vi "no ramp right.vi"() -> ()   [LabVIEW 2012, in "Omni2013.lvrbt"]
uses:
  Omni2013.lvrbt
  <vilib>/NXT/Hardware/Plugins/Tetrix 180 deg Servo/Tetrix180ServoAddress.ctl
  <vilib>/NXT/Hardware/Plugins/Tetrix DC Motor/TetrixDCMotorAddress.ctl
  <vilib>/NXT/Block Support/NXT_InputPort.ctl
  <vilib>/NXT/HiTechnic/HiTechnic Controls/HiTechnic Port.ctl
  <vilib>/NXT/Dual Mode Library/Waits/Wait_Num(msec).vi
  <vilib>/NXT/NXTIO Xnodes/NXTIONodeSubVIs/TETRIX IO Move Servos.vi
  <vilib>/NXT/NXTIO Xnodes/NXTIONodeSubVIs/TETRIX IO Move DC Motors.vi
  <vilib>/NXT/HiTechnic/HiTechnic Config/HiTechnic IRSeeker Mode1200Hz.vi
  <vilib>/NXT/Dual Mode Library/Sensors/Sonar_cm.vi
  <vilib>/NXT/Dual Mode Library/Display/drawNumber.vi
  <vilib>/NXT/HiTechnic/HiTechnic Read/HiTechnic IRSeeker Sensor_DC all.vi
  <vilib>/NXT/NXTIO Xnodes/AddressXNode/NXTIOAddress.xnode
  <vilib>/NXT/NXTIO Xnodes/NXTIOXNode/NXTIO.xnode
  <vilib>/NXT/Subs/LVHSConnector.ctl
  <vilib>/NXT/LegoClasses/BrickReference/BrickReference.lvclass
panel:
  in  "Rotation":dbl
  in  "Translation L&R":dbl
  in  "Translation U&D":dbl
  in  "Initial Time":dbl
  out "Enabled":bool
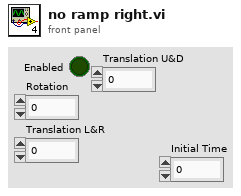
[diagram p1: front panel]
types:
  T1 = typedef "LVHSConnector.ctl" = refnum<class "BrickReference.lvclass">
  T2 = typedef "HiTechnic Port.ctl" = cluster{"Port":T3, "MUX Port":u8}
  T3 = typedef "NXT_InputPort.ctl" = u8
  T4 = typedef "TetrixDCMotorAddress.ctl" = i16
  T5 = cluster{"TetrixDCMotor":T4, "TetrixDCMotor 2":T4}
  T6 = typedef "Tetrix180ServoAddress.ctl" = i16
  T7 = cluster{"Direction (0-9)":i16, "Signal Strength (Array)":u8[]}
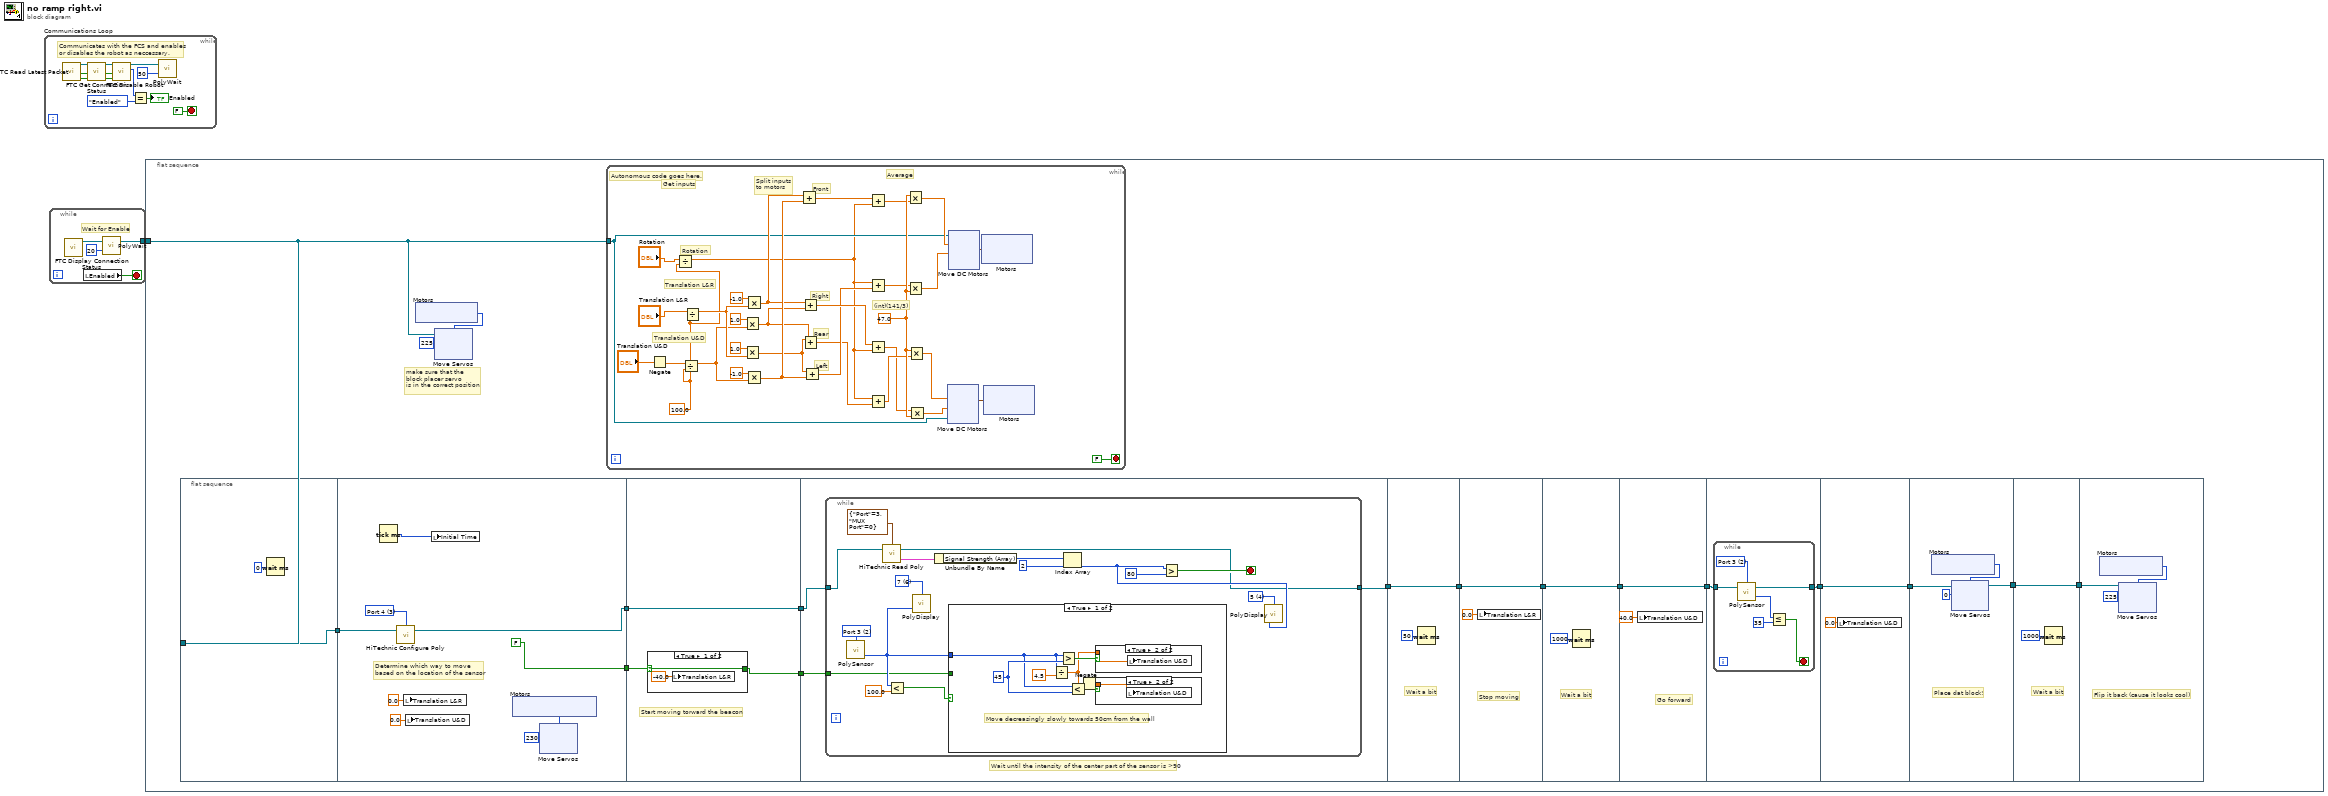
[diagram p0: block diagram]
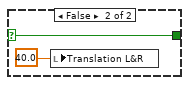
[diagram p2: hidden frame]
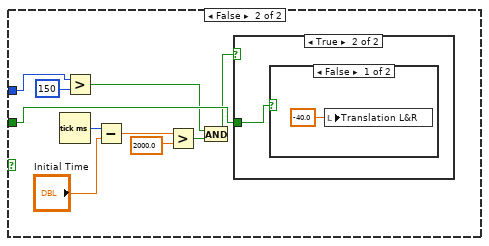
[diagram p5: hidden frame]
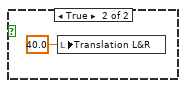
[diagram p7: hidden frame]
diagram:
  n1 = while "Communications Loop" {
    stop <- FALSE stop-if-true
    # "Communicates with the FCS and enables \nor disables the robot as neccessary."
    n2 = call <vilib>:"FTC Read Latest Packet.vi"() -> ("Packet Received?"=w11:bool, "Stopped?"=w10:bool, "NXT"=w13:T1)  [unwired: 6 in, 3 out]
    n3 = call <vilib>:"FTC Get Connection Status.vi"("Packet Received?"=w11, "Stopped?"=w10, "NXT"=w13) -> ("Online?"=w2:bool, "Stopped?"=w3:bool, "NXT"=w12:T1)  [unwired: 5 in]
    n4 = call <vilib>:"FTC Disable Robot.vi"("Online?"=w2, "Stopped?"=w3, "NXT"=w12) -> ("Enabled?"=w6:enum16{"Disabled", "Enabled"}, "NXT"=w8:T1)  [unwired: 3 in]
    n5 = Equal?(x=w6, y=enum16{"Disabled", "Enabled"}."Enabled") -> (x = y?=→"Enabled":bool)
    n6 = call-poly <vilib>:"PolyWait.vi"("Time (100 msec)"=u32 50 ("Time (msec)"), "NXT"=w8) -> ()  [unwired: 2 in, 1 out]
  }
  n7 = while {
    tunnel: [w15] -> w1
    stop <- w16 stop-if-true
    # "Wait for Enable"
    n8 = call <vilib>:"FTC Display Connection Status.vi"() -> ("NXT"=w14:T1)  [unwired: 11 in]
    n9 = local read "Enabled"() -> (w16:bool)
    n10 = call-poly <vilib>:"PolyWait.vi"("Time (100 msec)"=u32 20 ("Time (msec)"), "NXT"=w14) -> ("NXT"=w15:T1)  [unwired: 2 in]
  }
  n11 = flat-sequence {
    tunnel: w1 -> [w32]
    frame #0 {
      # "make sure that the \nblock placer servo \nis in the correct position"
      n12 = flat-sequence {
        tunnel: w32 -> [w44]
        tunnel: [w44] -> w18
        tunnel: [FALSE] -> w21
        tunnel: [w46] -> w20
        tunnel: w18 -> [w50]
        tunnel: [w64] -> w29
        tunnel: w21 -> [w63]
        tunnel: w20 -> [w64]
        tunnel: [w62] -> w19
        tunnel: w29 -> [w71]
        tunnel: [w70] -> w31
        tunnel: w19 -> [w69]
        tunnel: w31 -> [w111]
        tunnel: [w111] -> w30
        tunnel: [w112] -> w28
        tunnel: w30 -> [w112]
        tunnel: [w115] -> w22
        tunnel: w28 -> [w115]
        tunnel: w22 -> [w117]
        tunnel: [w117] -> w27
        tunnel: w27 -> [w119]
        tunnel: [w118] -> w26
        tunnel: w26 -> [w127]
        tunnel: [w127] -> w25
        tunnel: w25 -> [w129]
        tunnel: [w128] -> w24
        tunnel: w24 -> [w141]
        tunnel: [w141] -> w23
        tunnel: w23 -> [w142]
        frame #0 {
          n13 = Wait (ms)(milliseconds to wait=u32 0) -> ()  [unwired: 1 out]
        }
        frame #1 {
          w53 = T3 3 items=["Port 1", "Port 2", "Port 3", "Port 4"] ("Port")
          # "Determine which way to move \nbased on the location of the sensor"
          n14 = Tick Count (ms)() -> (millisecond timer value=w49:u32)
          n15 = call-poly <vilib>:"HiTechnic Configure Poly.vi"("NXT"=w50, "Port"=w53) -> ("NXT"=w46:T1)  [unwired: 2 in]
          n16 = local write "Translation L&R"(0.0 ("Translation L&R")) -> ()
          n17 = local write "Translation U&D"(0.0 ("Translation U&D")) -> ()
          n18 = local write "Initial Time"(w49) -> ()
          n19 = xnode "Motors"() -> ("Motor"=w48:T6)
          n20 = xnode "Move Servos"("Position 1"=u8 230, "Servos"=w48) -> ()  [unwired: 1 in, 1 out]
        }
        frame #2 {
          # "Start moving torward the beacon"
          n21 = case shown="True" w63 {
            selector: w63 -> [w65 w67]
            tunnel: [w65 w67] -> w62
            frame True {
              n22 = local write "Translation L&R"(-40.0 ("Translation L&R")) -> ()
            }
            frame False {
              n23 = local write "Translation L&R"(40.0 ("Translation L&R")) -> ()
            }
          }
        }
        frame #3 {
          # "Wait until the intensity of the center part of the sensor is >90"
          n24 = while {
            tunnel: w71 -> [w79]
            tunnel: [w77] -> w70
            tunnel: w69 -> [w72]
            stop <- w83 stop-if-true
            w76 = i16 6 items=["1", "2", "3", "4", "5", "6", "7", "8"] ("Line")
            w78 = T3 2 items=["Port 1", "Port 2", "Port 3", "Port 4"] ("Port (Port 4)")
            w82 = i16 4 items=["1", "2", "3", "4", "5", "6", "7", "8"] ("Line")
            n25 = call-poly <vilib>:"PolySensor.vi"("Port (Port 4)"=w78) -> ("Distance (cm)"=w74:i16)  [unwired: 2 in, 1 out]
            n26 = call-poly <vilib>:"HiTechnic Read Poly.vi"("NXT"=w79, "Port/MUX"=T2 {"Port"=3, "MUX Port"=0}) -> ("All Info"=w86:T7, "NXT"=w77:T1)  [unwired: 1 in]
            n27 = Less?(x=w74, y=100.0) -> (x < y?=w73:bool)
            n28 = call-poly <vilib>:"PolyDisplay.vi"("number"=w74, "Line"=w76) -> ()  [unwired: 2 in, 1 out]
            n29 = Unbundle By Name(w86) -> ("Signal Strength (Array)"=w85:u8[])
            n30 = case shown="True" w73 {
              tunnel: w74 -> [w90 w106]
              tunnel: w72 -> [_ w104]
              frame True {
                w92 = i16 45 ("y")
                # "Move decreasingly slowly towards 50cm from the wall"
                n31 = Divide(x=w90, y=4.5) -> (x/y=w89:dbl)
                n32 = Greater?(x=w90, y=w92) -> (0:w93:bool)
                n33 = Less?(x=w90, y=w92) -> (x < y?=w94:bool)
                n34 = Negate(x=w89) -> (-x=w88:dbl)
                n35 = case shown="True" w93 {
                  tunnel: w89 -> [_ w95]
                  frame False {
                  }
                  frame True {
                    n36 = local write "Translation U&D"(w95) -> ()
                  }
                }
                n37 = case shown="True" w94 {
                  tunnel: w88 -> [_ w96]
                  frame False {
                  }
                  frame True {
                    n38 = local write "Translation U&D"(w96) -> ()
                  }
                }
              }
              frame False {
                n39 = Tick Count (ms)() -> (millisecond timer value=w103:u32)
                n40 = Greater?(x=w106, y=i16 150) -> (0:w98:bool)
                n41 = Subtract(x=w103, y="Initial Time") -> (x-y=w101:dbl)
                n42 = Greater?(x=w101, y=2000.0) -> (0:w97:bool)
                n43 = And(x=w98, y=w97) -> (x .and. y?=w99:bool)
                n44 = case shown="True" w99 {
                  tunnel: w104 -> [_ w107]
                  frame False {
                  }
                  frame True {
                    n45 = case shown="False" w107 {
                      frame False {
                        n46 = local write "Translation L&R"(-40.0 ("Translation L&R")) -> ()
                      }
                      frame True {
                        n47 = local write "Translation L&R"(40.0 ("Translation L&R")) -> ()
                      }
                    }
                  }
                }
              }
            }
            n48 = Index Array(array=w85, index=2) -> (element=w81:u8)
            n49 = Greater?(x=w81, y=u8 80) -> (0:w83:bool)
            n50 = call-poly <vilib>:"PolyDisplay.vi"("number"=w81, "Line"=w82) -> ()  [unwired: 2 in, 1 out]
          }
        }
        frame #4 {
          # "Wait a bit"
          n51 = Wait (ms)(milliseconds to wait=u32 50) -> ()  [unwired: 1 out]
        }
        frame #5 {
          # "Stop moving"
          n52 = local write "Translation L&R"(0.0 ("Translation L&R")) -> ()
        }
        frame #6 {
          # "Wait a bit"
          n53 = Wait (ms)(milliseconds to wait=u32 1000) -> ()  [unwired: 1 out]
        }
        frame #7 {
          # "Go forward"
          n54 = local write "Translation U&D"(40.0 ("Translation U&D")) -> ()
        }
        frame #8 {
          n55 = while {
            tunnel: w119 -> [w122]
            tunnel: [w121] -> w118
            stop <- w123 stop-if-true
            w120 = T3 2 items=["Port 1", "Port 2", "Port 3", "Port 4"] ("Port (Port 4)")
            n56 = call-poly <vilib>:"PolySensor.vi"("NXT"=w122, "Port (Port 4)"=w120) -> ("Distance (cm)"=w125:i16, "NXT"=w121:T1)  [unwired: 1 in]
            n57 = Less Or Equal?(x=w125, y=i16 35) -> (x <= y?=w123:bool)
          }
        }
        frame #9 {
          n58 = local write "Translation U&D"(0.0 ("Translation U&D")) -> ()
        }
        frame #10 {
          # "Place dat block!"
          n59 = xnode "Motors"() -> ("Motor"=w131:T6)
          n60 = xnode "Move Servos"("Position 1"=u8 0, "Servos"=w131, "NXT"=w129) -> ("NXT"=w128:T1)
        }
        frame #11 {
          # "Wait a bit"
          n61 = Wait (ms)(milliseconds to wait=u32 1000) -> ()  [unwired: 1 out]
        }
        frame #12 {
          # "Flip it back (cause it looks cool)"
          n62 = xnode "Motors"() -> ("Motor"=w144:T6)
          n63 = xnode "Move Servos"("Position 1"=u8 225, "Servos"=w144, "NXT"=w142) -> ()  [unwired: 1 out]
        }
      }
      n64 = xnode "Motors"() -> ("Motor"=w34:T6)
      n65 = xnode "Move Servos"("Position 1"=u8 225, "Servos"=w34, "NXT"=w32) -> ()  [unwired: 1 out]
      n66 = while {
        tunnel: w32 -> [w158]
        stop <- FALSE stop-if-true
        w154 = 100.0 ("y")
        w185 = 47.0 ("y")
        # "Average"
        # "Left"
        # "Rear"
        # "Right"
        # "Front"
        # "(int)(141/3)"
        # "Split inputs to motors"
        # "Get inputs"
        # "Translation U&D"
        # "Rotation"
        # "Translation L&R"
        # "Autonomous code goes here."
        n67 = Negate(x="Translation U&D") -> (-x=w153:dbl)
        n68 = Divide(x="Rotation", y=w154) -> (x/y=w155:dbl)
        n69 = Divide(x=w153, y=w154) -> (x/y=w156:dbl)
        n70 = Divide(x="Translation L&R", y=w154) -> (x/y=w157:dbl)
        n71 = Multiply(x=1.0, y=w156) -> (x*y=w179:dbl)
        n72 = Multiply(x=1.0, y=w157) -> (x*y=w168:dbl)
        n73 = Multiply(x=-1.0, y=w157) -> (x*y=w167:dbl)
        n74 = Multiply(x=-1.0, y=w156) -> (x*y=w180:dbl)
        n75 = Add(x=w167, y=w180) -> (x+y=w164:dbl)
        n76 = Add(x=w167, y=w179) -> (x+y=w166:dbl)
        n77 = Add(x=w168, y=w179) -> (x+y=w163:dbl)
        n78 = Add(x=w168, y=w180) -> (x+y=w165:dbl)
        n79 = Add(x=w164, y=w155) -> (x+y=w183:dbl)
        n80 = Add(x=w155, y=w165) -> (x+y=w182:dbl)
        n81 = Add(x=w166, y=w155) -> (x+y=w181:dbl)
        n82 = Add(x=w155, y=w163) -> (x+y=w184:dbl)
        n83 = Multiply(x=w185, y=w183) -> (x*y=w174:dbl)
        n84 = Multiply(x=w182, y=w185) -> (x*y=w175:dbl)
        n85 = Multiply(x=w185, y=w184) -> (x*y=w178:dbl)
        n86 = Multiply(x=w181, y=w185) -> (x*y=w177:dbl)
        n87 = xnode "Motors"() -> ("Motor"=w173:cluster{"TetrixDCMotor":T4, "TetrixDCMotor":T4})
        n88 = xnode "Move DC Motors"("Power/Speed 2"=w175, "Power/Speed 1"=w174, "Motors"=w173, "NXT"=w158) -> ()  [unwired: 1 out]
        n89 = xnode "Motors"() -> ("Motor"=w176:cluster{"TetrixDCMotor":T4, "TetrixDCMotor":T4})
        n90 = xnode "Move DC Motors"("Power/Speed 2"=w177, "Power/Speed 1"=w178, "Motors"=w176, "NXT"=w158) -> ()  [unwired: 1 out]
      }
    }
  }
